vi "Get Status.vi"(8 "error in (no error)":errorcluster, 9 "Current Step":i32=1 caption="Step", 10 "Current Iteration":i32=1 caption="Iteration", 11 "Platform in":refnum<class "Platform.lvclass">) -> (0 "error out":errorcluster, 3 "Platform out":refnum<class "Platform.lvclass">)   [LabVIEW 2019, in "Platform.lvlib" / "Platform.lvclass"]
uses:
  Platform.lvclass
  Platform.lvclass/Platform.ctl
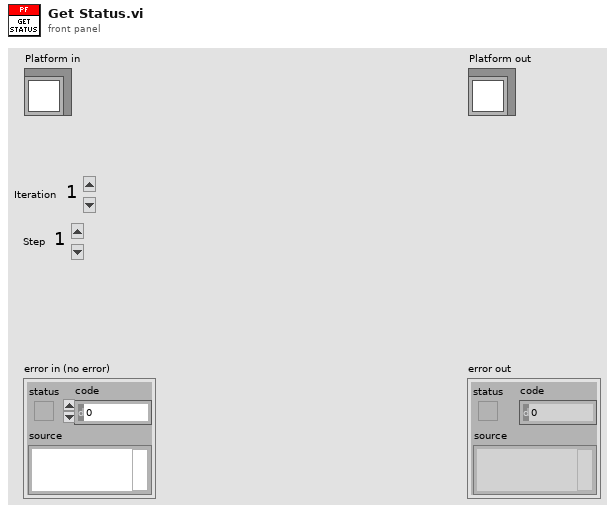
[diagram p1: front panel]
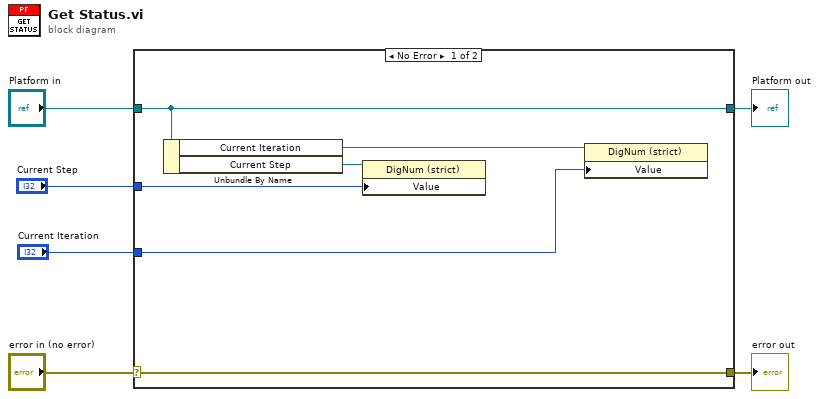
[diagram p0: block diagram]
diagram:
  n1 = case shown="No Error" "error in (no error)" {
    selector: "error in (no error)" -> [w12 w14]
    tunnel: [w12 w14] -> w5
    tunnel: [w11 w13] -> w3
    tunnel: "Platform in" -> [w11 w13]
    tunnel: "Current Step" -> [w9 _]
    tunnel: "Current Iteration" -> [w7 _]
    frame No Error {
      n2 = Unbundle By Name(w11) -> ("Current Iteration"=w8:refnum<vi>, "Current Step"=w10:refnum<vi>)
      n3 = property class="DigNum (strict)"(reference=w10, "Value"=w9) -> ()  [unwired: 1 in, 2 out]
      n4 = property class="DigNum (strict)"(reference=w8, "Value"=w7) -> ()  [unwired: 1 in, 2 out]
    }
    frame Error {
    }
  }
  "error out" <- w5
  "Platform out" <- w3
